vi "Main 2.3.vi"() -> ()   [LabVIEW 2022 SP3]
uses:
  <vilib>/MakerHub/LINX/Public/Utilities/Open Serial.vi
  <vilib>/MakerHub/LINX/Public/Sensors/Motion/Servo/Servo Open One Channel.vi
  Global 2 Horizontal old.vi
  Global 2 Horizontal.vi
  Global 4 Gripper old.vi
  Global 4 Gripper.vi
  Global 3 Vertical old.vi
  Global 3 Vertical.vi
  <vilib>/MakerHub/LINX/Public/Sensors/Motion/Servo/Servo Set Pulse Width One Channel.vi
  <vilib>/MakerHub/LINX/Public/Sensors/Motion/Servo/Servo Close One Channel.vi
  Global distance.vi
  Global 1 Base.vi
  Global 5 grid number.vi
  Global 6 Bool.vi
  Reading Red.vi
  Global Red Initial.vi
  Reading Green.vi
  Global Green Initial.vi
  Reading Blue.vi
  Global Blue Initial.vi
  Global Blue After Box.vi
  Global Green After Box.vi
  Global Red After Box.vi
  Colour Output.vi
  <vilib>/MakerHub/LINX/LMH-LINX.lvlib
  <vilib>/MakerHub/LINX/Public/Sensors/Motion/Servo/Servo.lvlib
panel:
  out "Numeric 6":dbl
  out "Numeric 5":dbl
  out "Numeric 4":dbl
  out "Numeric 3":dbl
  out "Numeric 2":dbl
  out "Numeric":dbl
  out "String":string
  out "Distance to Box 2":dbl
  out "Waveform Chart":dynamicdata(graph)
  out "Object detected":bool=TRUE
  out "Object not detected / Unreachable":bool=TRUE
  out "Base":i32
  out "Gripper":i32
  out "Vertical":i32
  out "Horzontal":i32
  out "Grid No":i32
  out "Starting":bool=TRUE
  out "Waiting":bool
  out "Over":bool=TRUE
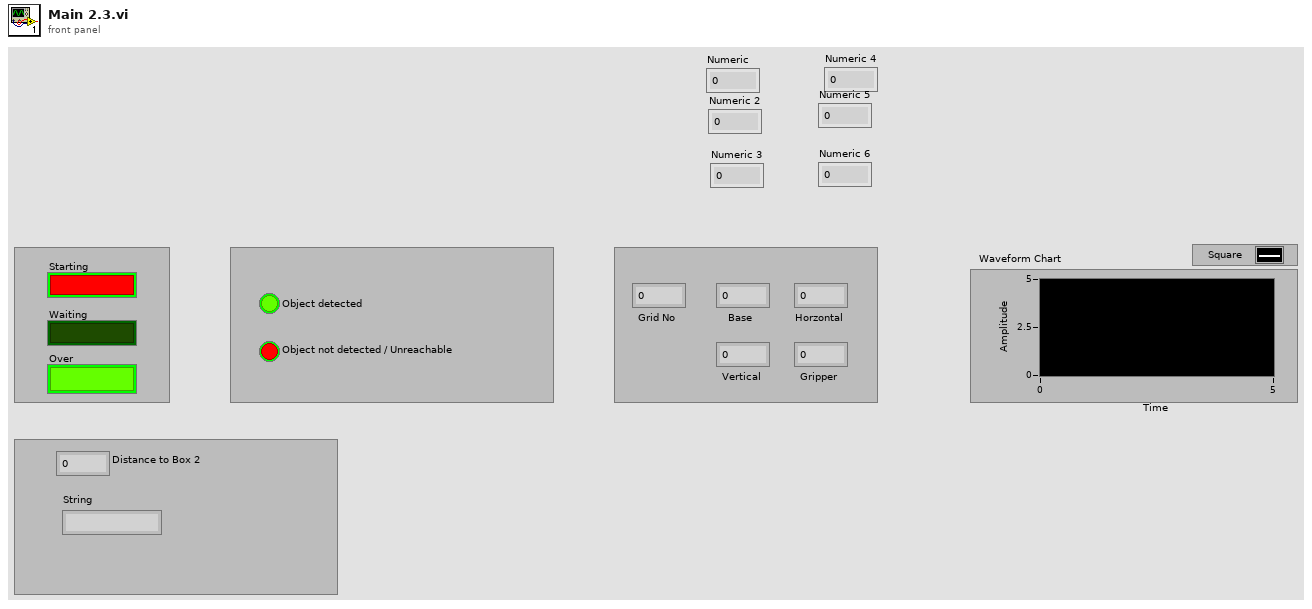
[diagram p1: front panel]
types:
  T1 = typedef "LMH-LINX.lvlib/LINX Ref.ctl" = cluster{"IO":T2, "Interface":T3, "LINX Device Config":T4}
  T2 = typedef "LMH-LINX.lvlib/Platform.ctl" = enum16{"Remote", "Local"}
  T3 = typedef "LMH-LINX.lvlib/Interface.ctl" = enum16{"Serial", "TCP"}
  T4 = typedef "LMH-LINX.lvlib/Device.lvlib/LINX Device Config.ctl" = cluster{"Interface":T3, "COM Port":refnum<visa-resource-name>, "TCP Configuration":T5, "Device Family":u8, "Device ID":u8, "Device Name":string, "TCP Ref":refnum<k5>, "Channels":T6}
  T5 = typedef "LMH-LINX.lvlib/Device.lvlib/TCP Config.ctl" = cluster{"IP Address":string, "Port":u16}
  T6 = typedef "LMH-LINX.lvlib/Channels.ctl" = cluster{"DI":u8[], "DO":u8[], "AI":u8[], "AO":u8[], "PWM":u8[], "QE":u8[], "UART":u8[], "I2C 2":u8[], "SPI":u8[], "CAN":u8[], "Servo":u8[], "AI Ref (V)":dbl, "AI Resolution (Bits)":u8, "AO Ref (V)":dbl, "AO Resolution (Bits)":u8}
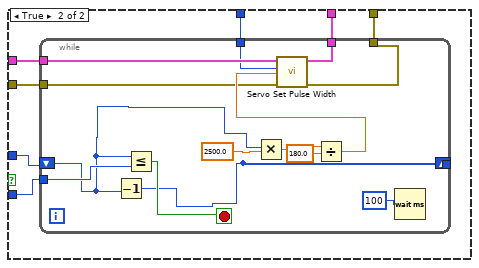
[diagram p2: hidden frame]
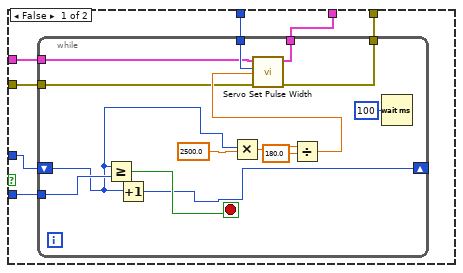
[diagram p3: hidden frame]
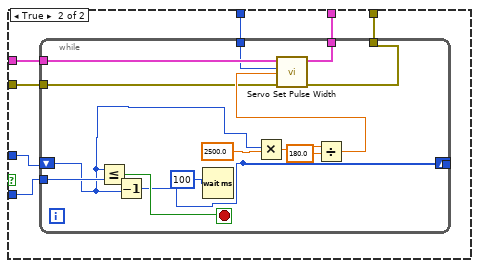
[diagram p4: hidden frame]
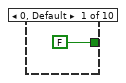
[diagram p5: hidden frame]
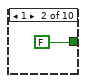
[diagram p6: hidden frame]
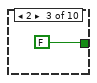
[diagram p7: hidden frame]
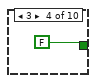
[diagram p8: hidden frame]
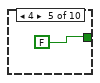
[diagram p9: hidden frame]
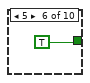
[diagram p10: hidden frame]
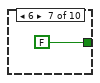
[diagram p11: hidden frame]
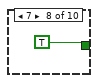
[diagram p12: hidden frame]
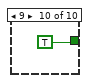
[diagram p13: hidden frame]
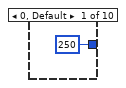
[diagram p14: hidden frame]
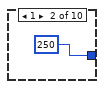
[diagram p15: hidden frame]
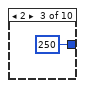
[diagram p16: hidden frame]
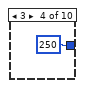
[diagram p17: hidden frame]
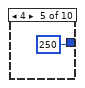
[diagram p18: hidden frame]
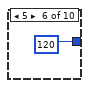
[diagram p19: hidden frame]
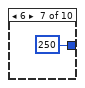
[diagram p20: hidden frame]
diagram:
  w8 = 11
  w6 = 10
  w3 = 9
  n1 = call-poly <vilib>:"Open.vi"("Serial Port"=refnum<visa-resource-name> "COM6") -> ("Error Out"=w9:errorcluster, "LINX Resource"=w10:T1)  [unwired: 8 in, 1 out]
  n2 = call-poly <vilib>:"Servo Open.vi"("Error In"=w9, "Servo Channel"=w3, "LINX Resource"=w10) -> ("Error Out"=w27:errorcluster, "LINX Resource"=w29:T1)  [unwired: 7 in]
  n3 = call-poly <vilib>:"Servo Open.vi"("Error In"=w9, "Servo Channel"=w6, "LINX Resource"=w10) -> ("Error Out"=w1:errorcluster, "LINX Resource"=w16:T1)  [unwired: 7 in]
  n4 = call-poly <vilib>:"Servo Open.vi"("Error In"=w9, "Servo Channel"=w8, "LINX Resource"=w10) -> ("Error Out"=w12:errorcluster, "LINX Resource"=w13:T1)  [unwired: 7 in]
  n5 = while {
    tunnel: w29 -> [w46]
    tunnel: [w44] -> w28
    tunnel: w27 -> [w48]
    tunnel: [w45] -> w26
    tunnel: w3 -> [w49]
    tunnel: w16 -> [w53]
    tunnel: [w52] -> w15
    tunnel: [w42] -> w14
    tunnel: w13 -> [w40]
    tunnel: w12 -> [w39]
    tunnel: [w41] -> w11
    tunnel: w8 -> [w43]
    tunnel: [w43] -> w7
    tunnel: w6 -> [w54]
    tunnel: [w54] -> w5
    tunnel: [w49] -> w4
    tunnel: [w51] -> w2
    tunnel: w1 -> [w50]
    stop <- w37 stop-if-true
    # "Arm servo control"
    n6 = global read "Global 2 Horizontal old.vi" "Numeric"() -> (w32:i32)
    n7 = global read "Global 2 Horizontal.vi" "Numeric"() -> (w31:i32)
    n8 = global read "Global 3 Vertical old.vi" "Numeric"() -> (w34:i32)
    n9 = global read "Global 3 Vertical.vi" "Numeric"() -> (w33:i32)
    n10 = global read "Global 4 Gripper old.vi" "Numeric"() -> (w36:i32)
    n11 = global read "Global 4 Gripper.vi" "Numeric"() -> (w35:i32)
    n12 = Greater?(x=w32, y=w31) -> (0:w47:bool)
    n13 = case shown="True" w47 {
      tunnel: w32 -> [w103 w124]
      tunnel: w31 -> [w104 w125]
      tunnel: w49 -> [w102 w121]
      tunnel: [w101 w123] -> w45
      tunnel: w48 -> [w100 w122]
      tunnel: w46 -> [w99 w119]
      tunnel: [w98 w120] -> w44
      frame False {
        n14 = while {
          tunnel: w104 -> [w115]
          shift-right: [w116] -> _
          shift-left: w103 -> [w108]
          tunnel: w102 -> [w110]
          tunnel: [w109] -> w98
          tunnel: [w107] -> w101
          tunnel: w100 -> [w106]
          tunnel: w99 -> [w105]
          stop <- w118 stop-if-true
          n15 = Greater Or Equal?(x=w108, y=w115) -> (x >= y?=w118:bool)
          n16 = Increment(x=w108) -> (x+1=w116:i32)
          n17 = Multiply(x=w108, y=2500.0) -> (x*y=w113:dbl)
          n18 = Divide(x=w113, y=180.0) -> (x/y=w114:dbl)
          n19 = call-poly <vilib>:"Servo Set Pulse Width.vi"("Error In"=w106, "Pulse Width (uS)"=w114, "Servo Channel"=w110, "LINX Resource"=w105) -> ("Error Out"=w107:errorcluster, "LINX Resource"=w109:T1)  [unwired: 6 in]
          n20 = Wait (ms)(milliseconds to wait=u32 100 ("millisecond timer value")) -> ()  [unwired: 1 out]
        }
      }
      frame True {
        n21 = while {
          tunnel: w125 -> [w139]
          tunnel: [w138] -> _
          shift-right: [w128] -> _
          shift-left: w124 -> [w130]
          tunnel: [w128] -> _
          tunnel: [w132] -> w123
          tunnel: w122 -> [w131]
          tunnel: w121 -> [w129]
          tunnel: [w127] -> w120
          tunnel: w119 -> [w126]
          stop <- w138 stop-if-true
          n22 = Less Or Equal?(x=w130, y=w139) -> (x <= y?=w138:bool)
          n23 = Decrement(x=w130) -> (x-1=w128:i32)
          n24 = Multiply(x=w130, y=2500.0) -> (x*y=w135:dbl)
          n25 = Divide(x=w135, y=180.0) -> (x/y=w136:dbl)
          n26 = call-poly <vilib>:"Servo Set Pulse Width.vi"("Error In"=w131, "Pulse Width (uS)"=w136, "Servo Channel"=w129, "LINX Resource"=w126) -> ("Error Out"=w132:errorcluster, "LINX Resource"=w127:T1)  [unwired: 6 in]
          n27 = Wait (ms)(milliseconds to wait=u32 100 ("millisecond timer value")) -> ()  [unwired: 1 out]
        }
      }
    }
    n28 = Greater?(x=w34, y=w33) -> (0:w55:bool)
    n29 = Greater?(x=w36, y=w35) -> (0:w38:bool)
    n30 = case shown="False" w55 {
      tunnel: w34 -> [w145 w166]
      tunnel: w33 -> [w146 w167]
      tunnel: w54 -> [w144 w161]
      tunnel: w53 -> [w143 w163]
      tunnel: [w142 w164] -> w52
      tunnel: [w141 w165] -> w51
      tunnel: w50 -> [w140 w162]
      frame False {
        n31 = while {
          tunnel: w146 -> [w157]
          shift-right: [w158] -> _
          shift-left: w145 -> [w149]
          tunnel: w144 -> [w152]
          tunnel: w143 -> [w151]
          tunnel: [w150] -> w142
          tunnel: [w148] -> w141
          tunnel: w140 -> [w147]
          stop <- w160 stop-if-true
          n32 = Greater Or Equal?(x=w149, y=w157) -> (x >= y?=w160:bool)
          n33 = Increment(x=w149) -> (x+1=w158:i32)
          n34 = Wait (ms)(milliseconds to wait=u32 100 ("millisecond timer value")) -> ()  [unwired: 1 out]
          n35 = Multiply(x=w149, y=2500.0) -> (x*y=w155:dbl)
          n36 = Divide(x=w155, y=180.0) -> (x/y=w156:dbl)
          n37 = call-poly <vilib>:"Servo Set Pulse Width.vi"("Error In"=w147, "Pulse Width (uS)"=w156, "Servo Channel"=w152, "LINX Resource"=w151) -> ("Error Out"=w148:errorcluster, "LINX Resource"=w150:T1)  [unwired: 6 in]
        }
      }
      frame True {
        n38 = while {
          tunnel: w167 -> [w181]
          shift-right: [w178] -> _
          shift-left: w166 -> [w169]
          tunnel: [w178] -> _
          tunnel: [w173] -> w165
          tunnel: [w172] -> w164
          tunnel: w163 -> [w171]
          tunnel: w162 -> [w170]
          tunnel: w161 -> [w168]
          stop <- w180 stop-if-true
          n39 = Less Or Equal?(x=w169, y=w181) -> (x <= y?=w180:bool)
          n40 = Decrement(x=w169) -> (x-1=w178:i32)
          n41 = Wait (ms)(milliseconds to wait=u32 100 ("millisecond timer value")) -> ()  [unwired: 1 out]
          n42 = Multiply(x=w169, y=2500.0) -> (x*y=w176:dbl)
          n43 = Divide(x=w176, y=180.0) -> (x/y=w177:dbl)
          n44 = call-poly <vilib>:"Servo Set Pulse Width.vi"("Error In"=w170, "Pulse Width (uS)"=w177, "Servo Channel"=w168, "LINX Resource"=w171) -> ("Error Out"=w173:errorcluster, "LINX Resource"=w172:T1)  [unwired: 6 in]
        }
      }
    }
    n45 = case shown="False" w38 {
      tunnel: w36 -> [w61 w82]
      tunnel: w35 -> [w62 w83]
      tunnel: w43 -> [w60 w77]
      tunnel: w40 -> [w59 w79]
      tunnel: [w58 w80] -> w42
      tunnel: [w57 w81] -> w41
      tunnel: w39 -> [w56 w78]
      frame False {
        n46 = while {
          tunnel: w62 -> [w73]
          shift-right: [w74] -> _
          shift-left: w61 -> [w65]
          tunnel: w60 -> [w68]
          tunnel: w59 -> [w67]
          tunnel: [w66] -> w58
          tunnel: [w64] -> w57
          tunnel: w56 -> [w63]
          stop <- w76 stop-if-true
          n47 = Greater Or Equal?(x=w65, y=w73) -> (x >= y?=w76:bool)
          n48 = Increment(x=w65) -> (x+1=w74:i32)
          n49 = Multiply(x=w65, y=2500.0) -> (x*y=w71:dbl)
          n50 = Divide(x=w71, y=180.0) -> (x/y=w72:dbl)
          n51 = call-poly <vilib>:"Servo Set Pulse Width.vi"("Error In"=w63, "Pulse Width (uS)"=w72, "Servo Channel"=w68, "LINX Resource"=w67) -> ("Error Out"=w64:errorcluster, "LINX Resource"=w66:T1)  [unwired: 6 in]
          n52 = Wait (ms)(milliseconds to wait=u32 100 ("millisecond timer value")) -> ()  [unwired: 1 out]
        }
      }
      frame True {
        n53 = while {
          tunnel: w83 -> [w97]
          shift-right: [w94] -> _
          shift-left: w82 -> [w85]
          tunnel: [w94] -> _
          tunnel: [w89] -> w81
          tunnel: [w88] -> w80
          tunnel: w79 -> [w87]
          tunnel: w78 -> [w86]
          tunnel: w77 -> [w84]
          stop <- w96 stop-if-true
          n54 = Decrement(x=w85) -> (x-1=w94:i32)
          n55 = Less Or Equal?(x=w85, y=w97) -> (x <= y?=w96:bool)
          n56 = Multiply(x=w85, y=2500.0) -> (x*y=w92:dbl)
          n57 = Divide(x=w92, y=180.0) -> (x/y=w93:dbl)
          n58 = call-poly <vilib>:"Servo Set Pulse Width.vi"("Error In"=w86, "Pulse Width (uS)"=w93, "Servo Channel"=w84, "LINX Resource"=w87) -> ("Error Out"=w89:errorcluster, "LINX Resource"=w88:T1)  [unwired: 6 in]
          n59 = Wait (ms)(milliseconds to wait=u32 100 ("millisecond timer value")) -> ()  [unwired: 1 out]
        }
      }
    }
    n60 = local read "Over"() -> (w37:bool)
  }
  n61 = call-poly <vilib>:"Servo Close.vi"("Error In"=w26, "Servo Channel"=w4, "LINX Resource"=w28) -> ("Error Out"=w23:errorcluster, "LINX Resource"=w24:T1)  [unwired: 7 in]
  n62 = call-poly <vilib>:"Servo Close.vi"("Error In"=w2, "Servo Channel"=w5, "LINX Resource"=w15) -> ("Error Out"=w20:errorcluster, "LINX Resource"=w21:T1)  [unwired: 7 in]
  n63 = call-poly <vilib>:"Servo Close.vi"("Error In"=w11, "Servo Channel"=w7, "LINX Resource"=w14) -> ("Error Out"=w17:errorcluster, "LINX Resource"=w18:T1)  [unwired: 7 in]
  n64 = call <vilib>:"Close.vi"("Error In"=w23, "LINX Resource"=w24) -> ("Error Out"=w25:errorcluster)  [unwired: 9 in]
  n65 = call <vilib>:"Close.vi"("Error In"=w20, "LINX Resource"=w21) -> ("Error Out"=w22:errorcluster)  [unwired: 9 in]
  n66 = call <vilib>:"Close.vi"("Error In"=w17, "LINX Resource"=w18) -> ("Error Out"=w19:errorcluster)  [unwired: 9 in]
  n67 = call <vilib>:"Simple Error Handler.vi"("error in (no error)"=w25) -> ()  [unwired: 4 in, 5 out]
  n68 = call <vilib>:"Simple Error Handler.vi"("error in (no error)"=w19) -> ()  [unwired: 4 in, 5 out]
  n69 = call <vilib>:"Simple Error Handler.vi"("error in (no error)"=w22) -> ()  [unwired: 4 in, 5 out]
  n70 = while {
    stop <- w184 stop-if-true
    # "Base servo control"
    # "Amplitude"
    # "Frequency"
    # "Offset"
    n71 = global read "Global 1 Base.vi" "Numeric"() -> (w183:i32)
    n72 = Divide(x=w183, y=36) -> (x/y=w192:dbl)
    n73 = Add(x=w192, y=5.0) -> (x+y=w191:dbl)
    n74 = call "Simulate Signal"("Offset"=2.5, "Duty Cycle (%)"=w191, "Frequency"=50.0, "Amplitude"=2.5) -> ("Square"=w182:dynamicdata)  [unwired: 10 in, 1 out]
    "Waveform Chart" <- w182
    n75 = call "DAQ Assistant"("data"=w182, "timeout (s)"=5.0) -> ()  [unwired: 15 in, 3 out]
    n76 = local read "Over"() -> (w184:bool)
  }
  n77 = while {
    stop <- w194 stop-if-true
    # "Ultrasonic sensor"
    n78 = global read "Global distance.vi" "Numeric"() -> (→"Distance to Box 2":dbl)
    n79 = call "ultrasonic.vi"() -> ()  [unwired: 12 in]
    n80 = local read "Over"() -> (w194:bool)
  }
  n81 = flat-sequence {
    frame #0 {
      # "Initiate"
      n82 = global write "Global 1 Base.vi" "Numeric"(250 ("Numeric")) -> ()
      n83 = global write "Global distance.vi" "Numeric"(0.0 ("Numeric")) -> ()
      n84 = global write "Global 4 Gripper.vi" "Numeric"(60 ("Numeric")) -> ()
      n85 = global write "Global 2 Horizontal.vi" "Numeric"(50 ("Numeric")) -> ()
      n86 = global write "Global 3 Vertical.vi" "Numeric"(160 ("Numeric")) -> ()
      n87 = Wait (ms)(milliseconds to wait=u32 3000 ("millisecond timer value")) -> ()  [unwired: 1 out]
      "Object not detected / Unreachable" <- FALSE
      "Object detected" <- FALSE
      "Over" <- FALSE
      "Waiting" <- FALSE
      "Starting" <- TRUE
    }
    frame #1 {
      # "Initial position"
      n88 = global write "Global 3 Vertical.vi" "Numeric"(160 ("Numeric")) -> ()
      n89 = global write "Global 4 Gripper.vi" "Numeric"(50 ("Numeric")) -> ()
      n90 = global write "Global 1 Base.vi" "Numeric"(250 ("Numeric")) -> ()
      n91 = global write "Global 2 Horizontal.vi" "Numeric"(60 ("Numeric")) -> ()
      n92 = local write "Starting"(FALSE) -> ()
      n93 = Wait (ms)(milliseconds to wait=u32 5000 ("millisecond timer value")) -> ()  [unwired: 1 out]
    }
    frame #2 {
      n94 = global read "Global 4 Gripper.vi" "Numeric"() -> (w213:i32)
      n95 = global read "Global 2 Horizontal.vi" "Numeric"() -> (w215:i32)
      n96 = global read "Global 3 Vertical.vi" "Numeric"() -> (w214:i32)
      n97 = global write "Global 2 Horizontal old.vi" "Numeric"(w215) -> ()
      n98 = global write "Global 3 Vertical old.vi" "Numeric"(w214) -> ()
      n99 = global write "Global 4 Gripper old.vi" "Numeric"(w213) -> ()
      n100 = Wait (ms)(milliseconds to wait=u32 1000 ("millisecond timer value")) -> ()  [unwired: 1 out]
    }
    frame #3 {
      # "Ready position"
      n101 = global write "Global 2 Horizontal.vi" "Numeric"(90 ("Numeric")) -> ()
      n102 = Wait (ms)(milliseconds to wait=u32 3000 ("millisecond timer value")) -> ()  [unwired: 1 out]
    }
    frame #4 {
      n103 = global write "Global 3 Vertical.vi" "Numeric"(120 ("Numeric")) -> ()
      n104 = Wait (ms)(milliseconds to wait=u32 3000 ("millisecond timer value")) -> ()  [unwired: 1 out]
    }
    frame #5 {
      n105 = global read "Global 2 Horizontal.vi" "Numeric"() -> (w222:i32)
      n106 = global read "Global 3 Vertical.vi" "Numeric"() -> (w221:i32)
      n107 = global write "Global 2 Horizontal old.vi" "Numeric"(w222) -> ()
      n108 = global write "Global 3 Vertical old.vi" "Numeric"(w221) -> ()
      n109 = Wait (ms)(milliseconds to wait=u32 1000 ("millisecond timer value")) -> ()  [unwired: 1 out]
    }
    frame #6 {
      # "Run .py"
      n110 = Open Python Session(python version="3.9" ("Python version"), python path=path "C:/Users/ASUS/AppData/Local/Programs/Python/Python39/python.exe" ("Python path")) -> (session out=w225:refnum<k35>, error out=w224:errorcluster)  [unwired: 1 in]
      n111 = node "Python Node"(w225, path "C:/Users/ASUS/Desktop/Project/grid.py" ("module path"), "detect_grid" ("function name"), w224) -> (w228:refnum<k35>, w227:errorcluster)  [unwired: 2 in, 2 out]
      n112 = Close Python Session(session in=w228, error in=w227) -> ()  [unwired: 1 out]
    }
    frame #7 {
      # "Read grid no. from .txt"
      n113 = Read from Text File(file (use dialog)=path "C:/Users/ASUS/Desktop/Project/grid_value.txt") -> (text=w232:string)  [unwired: 3 in, 3 out]
      n114 = Fract/Exp String To Number(string=w232) -> (number=w231:dbl)  [unwired: 3 in, 1 out]
      "Grid No" <- w231
      n115 = global write "Global 5 grid number.vi" "Numeric"(w231) -> ()
    }
    frame #8 {
      # "Grid selection"
      n116 = global read "Global 5 grid number.vi" "Numeric"() -> (w236:i32)
      n117 = case shown="8" w236 {
        tunnel: [FALSE FALSE FALSE FALSE FALSE TRUE FALSE TRUE FALSE TRUE] -> w235
        frame 0, Default {
        }
        frame 1 {
        }
        frame 2 {
        }
        frame 3 {
        }
        frame 4 {
        }
        frame 5 {
        }
        frame 6 {
        }
        frame 7 {
        }
        frame 8 {
        }
        frame 9 {
        }
      }
      n118 = global write "Global 6 Bool.vi" "Boolean"(w235) -> ()
      n119 = Wait (ms)(milliseconds to wait=u32 3000 ("millisecond timer value")) -> ()  [unwired: 1 out]
    }
    frame #9 {
      n120 = global read "Global 6 Bool.vi" "Boolean"() -> (w248:bool)
      n121 = Not(x=w248) -> (.not. x?=w247:bool)
      n122 = local write "Object not detected / Unreachable"(w247) -> ()
      n123 = local write "Object detected"(w248) -> ()
    }
    frame #10 {
      # "Get angles"
      n124 = global read "Global 5 grid number.vi" "Numeric"() -> (w251:i32)
      n125 = case shown="7" w251 {
        tunnel: [250 250 250 250 250 120 250 160 250 65] -> w250
        frame 0, Default {
        }
        frame 1 {
        }
        frame 2 {
        }
        frame 3 {
        }
        frame 4 {
        }
        frame 5 {
        }
        frame 6 {
        }
        frame 7 {
        }
        frame 8 {
        }
        frame 9 {
        }
      }
      "Base" <- w250
      n126 = global write "Global 1 Base.vi" "Numeric"(w250) -> ()
      n127 = Wait (ms)(milliseconds to wait=u32 3000 ("millisecond timer value")) -> ()  [unwired: 1 out]
    }
    frame #11 {
      # "Get angles"
      n128 = global read "Global 5 grid number.vi" "Numeric"() -> (w263:i32)
      n129 = case shown="8" w263 {
        tunnel: [0 0 0 0 0 120 0 120 0 120] -> w264
        frame 0, Default {
        }
        frame 1 {
        }
        frame 2 {
        }
        frame 3 {
        }
        frame 4 {
        }
        frame 5 {
        }
        frame 6 {
        }
        frame 7 {
        }
        frame 8 {
        }
        frame 9 {
        }
      }
      "Gripper" <- w264
      n130 = global write "Global 4 Gripper.vi" "Numeric"(w264) -> ()
      n131 = Wait (ms)(milliseconds to wait=u32 3000 ("millisecond timer value")) -> ()  [unwired: 1 out]
    }
    frame #12 {
      n132 = global read "Global 4 Gripper.vi" "Numeric"() -> (w275:i32)
      n133 = global write "Global 4 Gripper old.vi" "Numeric"(w275) -> ()
    }
    frame #13 {
      # "Get angles"
      n134 = global read "Global 5 grid number.vi" "Numeric"() -> (w278:i32)
      n135 = case shown="8" w278 {
        tunnel: [160 160 160 160 160 150 160 140 160 140] -> w277
        frame 0, Default {
        }
        frame 1 {
        }
        frame 2 {
        }
        frame 3 {
        }
        frame 4 {
        }
        frame 5 {
        }
        frame 6 {
        }
        frame 7 {
        }
        frame 8 {
        }
        frame 9 {
        }
      }
      "Vertical" <- w277
      n136 = global write "Global 3 Vertical.vi" "Numeric"(w277) -> ()
      n137 = Wait (ms)(milliseconds to wait=u32 3000 ("millisecond timer value")) -> ()  [unwired: 1 out]
    }
    frame #14 {
      n138 = global read "Global 3 Vertical.vi" "Numeric"() -> (w289:i32)
      n139 = global write "Global 3 Vertical old.vi" "Numeric"(w289) -> ()
    }
    frame #15 {
      # "Get angles"
      n140 = global read "Global 5 grid number.vi" "Numeric"() -> (w291:i32)
      n141 = case shown="9" w291 {
        tunnel: [60 60 60 60 60 125 60 118 60 115] -> w292
        frame 0, Default {
        }
        frame 1 {
        }
        frame 2 {
        }
        frame 3 {
        }
        frame 4 {
        }
        frame 5 {
        }
        frame 6 {
        }
        frame 7 {
        }
        frame 8 {
        }
        frame 9 {
        }
      }
      "Horzontal" <- w292
      n142 = global write "Global 2 Horizontal.vi" "Numeric"(w292) -> ()
      n143 = Wait (ms)(milliseconds to wait=u32 3000 ("millisecond timer value")) -> ()  [unwired: 1 out]
    }
    frame #16 {
      n144 = global read "Global 2 Horizontal.vi" "Numeric"() -> (w304:i32)
      n145 = global write "Global 2 Horizontal old.vi" "Numeric"(w304) -> ()
      n146 = Wait (ms)(milliseconds to wait=u32 3000 ("millisecond timer value")) -> ()  [unwired: 1 out]
    }
    frame #17 {
      n147 = global read "Global 6 Bool.vi" "Boolean"() -> (w305:bool)
      n148 = case shown="False" w305 {
        frame False {
          n149 = flat-sequence {
            frame #0 {
              n150 = global read "Global 6 Bool.vi" "Boolean"() -> (w306:bool)
              n151 = local write "Object not detected / Unreachable"(w306) -> ()
            }
            frame #1 {
              n152 = local write "Waiting"(TRUE) -> ()
              n153 = Wait (ms)(milliseconds to wait=u32 10000) -> ()  [unwired: 1 out]
            }
            frame #2 {
              n154 = call "Buzzer.vi"() -> ()  [unwired: 12 in]
            }
            frame #3 {
              n155 = local write "Waiting"(FALSE) -> ()
              n156 = Wait (ms)(milliseconds to wait=u32 3000) -> ()  [unwired: 1 out]
              n157 = local write "Over"(TRUE) -> ()
            }
          }
        }
        frame True {
          n158 = flat-sequence {
            frame #0 {
              # "Close the gripper"
              n159 = global write "Global 4 Gripper.vi" "Numeric"(50) -> ()
              n160 = Wait (ms)(milliseconds to wait=u32 5000) -> ()  [unwired: 1 out]
            }
            frame #1 {
              n161 = global read "Global 4 Gripper.vi" "Numeric"() -> (w315:i32)
              n162 = global write "Global 4 Gripper old.vi" "Numeric"(w315) -> ()
              n163 = Wait (ms)(milliseconds to wait=u32 5000) -> ()  [unwired: 1 out]
            }
            frame #2 {
              n164 = global write "Global 2 Horizontal.vi" "Numeric"(65) -> ()
              n165 = Wait (ms)(milliseconds to wait=u32 5000 ("millisecond timer value")) -> ()  [unwired: 1 out]
            }
            frame #3 {
              # "Pick up the box"
              n166 = global write "Global 3 Vertical.vi" "Numeric"(170) -> ()
              n167 = Wait (ms)(milliseconds to wait=u32 5000 ("millisecond timer value")) -> ()  [unwired: 1 out]
            }
            frame #4 {
              n168 = global read "Global 2 Horizontal.vi" "Numeric"() -> (w322:i32)
              n169 = global read "Global 3 Vertical.vi" "Numeric"() -> (w321:i32)
              n170 = global write "Global 2 Horizontal old.vi" "Numeric"(w322) -> ()
              n171 = global write "Global 3 Vertical old.vi" "Numeric"(w321) -> ()
              n172 = Wait (ms)(milliseconds to wait=u32 2000 ("millisecond timer value")) -> ()  [unwired: 1 out]
            }
            frame #5 {
              n173 = call "Colour.vi"() -> ()  [unwired: 12 in]
            }
            frame #6 {
              n174 = global read "Reading Red.vi" "Numeric"() -> (w325:dbl)
              "Numeric" <- w325
              n175 = global read "Reading Green.vi" "Numeric"() -> (w324:dbl)
              "Numeric 2" <- w324
              n176 = global read "Reading Blue.vi" "Numeric"() -> (w323:dbl)
              "Numeric 3" <- w323
              n177 = global write "Global Red Initial.vi" "Numeric"(w325) -> ()
              n178 = global write "Global Green Initial.vi" "Numeric"(w324) -> ()
              n179 = global write "Global Blue Initial.vi" "Numeric"(w323) -> ()
            }
            frame #7 {
              n180 = global write "Global 1 Base.vi" "Numeric"(-70 ("Numeric")) -> ()
              n181 = Wait (ms)(milliseconds to wait=u32 1000 ("millisecond timer value")) -> ()  [unwired: 1 out]
            }
            frame #8 {
              n182 = global write "Global 3 Vertical.vi" "Numeric"(160) -> ()
              n183 = Wait (ms)(milliseconds to wait=u32 1000 ("millisecond timer value")) -> ()  [unwired: 1 out]
            }
            frame #9 {
              n184 = global read "Global 3 Vertical.vi" "Numeric"() -> (w330:i32)
              n185 = global write "Global 3 Vertical old.vi" "Numeric"(w330) -> ()
            }
            frame #10 {
              n186 = call "Colour.vi"() -> ()  [unwired: 12 in]
            }
            frame #11 {
              n187 = global read "Reading Red.vi" "Numeric"() -> (w333:dbl)
              "Numeric 4" <- w333
              n188 = global read "Reading Green.vi" "Numeric"() -> (w332:dbl)
              "Numeric 5" <- w332
              n189 = global read "Reading Blue.vi" "Numeric"() -> (w331:dbl)
              "Numeric 6" <- w331
              n190 = global write "Global Red After Box.vi" "Numeric"(w333) -> ()
              n191 = global write "Global Green After Box.vi" "Numeric"(w332) -> ()
              n192 = global write "Global Blue After Box.vi" "Numeric"(w331) -> ()
            }
            frame #12 {
              n193 = global write "Global 4 Gripper.vi" "Numeric"(50) -> ()
              n194 = Wait (ms)(milliseconds to wait=u32 5000 ("millisecond timer value")) -> ()  [unwired: 1 out]
            }
            frame #13 {
              n195 = call "ColourCheck.vi"() -> ()  [unwired: 12 in]
            }
            frame #14 {
              n196 = global read "Colour Output.vi" "String"() -> (→"String":string)
            }
            frame #15 {
              n197 = global read "Colour Output.vi" "String"() -> (w337:string)
              n198 = case shown="\"red\", Default" w337 {
                frame "red", Default {
                  n199 = flat-sequence {
                    frame #0 {
                      n200 = global write "Global 1 Base.vi" "Numeric"(-70 ("Numeric")) -> ()
                      n201 = Wait (ms)(milliseconds to wait=u32 1000 ("millisecond timer value")) -> ()  [unwired: 1 out]
                    }
                    frame #1 {
                      n202 = global write "Global 3 Vertical.vi" "Numeric"(160) -> ()
                      n203 = Wait (ms)(milliseconds to wait=u32 1000 ("millisecond timer value")) -> ()  [unwired: 1 out]
                    }
                    frame #2 {
                      n204 = Wait (ms)(milliseconds to wait=u32 5000 ("millisecond timer value")) -> ()  [unwired: 1 out]
                      n205 = global write "Global 2 Horizontal.vi" "Numeric"(110) -> ()
                    }
                    frame #3 {
                      n206 = global read "Global 2 Horizontal.vi" "Numeric"() -> (w345:i32)
                      n207 = global read "Global 3 Vertical.vi" "Numeric"() -> (w344:i32)
                      n208 = global write "Global 2 Horizontal old.vi" "Numeric"(w345) -> ()
                      n209 = global write "Global 3 Vertical old.vi" "Numeric"(w344) -> ()
                    }
                    frame #4 {
                      n210 = global write "Global 4 Gripper.vi" "Numeric"(120) -> ()
                      n211 = Wait (ms)(milliseconds to wait=u32 5000 ("millisecond timer value")) -> ()  [unwired: 1 out]
                    }
                    frame #5 {
                      n212 = global read "Global 4 Gripper.vi" "Numeric"() -> (w349:i32)
                      n213 = global write "Global 4 Gripper old.vi" "Numeric"(w349) -> ()
                      n214 = Wait (ms)(milliseconds to wait=u32 3000) -> ()  [unwired: 1 out]
                    }
                    frame #6 {
                      n215 = global write "Global 3 Vertical.vi" "Numeric"(180) -> ()
                      n216 = Wait (ms)(milliseconds to wait=u32 5000 ("millisecond timer value")) -> ()  [unwired: 1 out]
                    }
                    frame #7 {
                      n217 = Wait (ms)(milliseconds to wait=u32 5000 ("millisecond timer value")) -> ()  [unwired: 1 out]
                      n218 = global write "Global 2 Horizontal.vi" "Numeric"(70) -> ()
                    }
                    frame #8 {
                      n219 = global read "Global 2 Horizontal.vi" "Numeric"() -> (w354:i32)
                      n220 = global read "Global 3 Vertical.vi" "Numeric"() -> (w355:i32)
                      n221 = global write "Global 2 Horizontal old.vi" "Numeric"(w354) -> ()
                      n222 = global write "Global 3 Vertical old.vi" "Numeric"(w355) -> ()
                    }
                    frame #9 {
                      n223 = global write "Global 4 Gripper.vi" "Numeric"(60) -> ()
                    }
                  }
                }
                frame "green" {
                  n224 = flat-sequence {
                    frame #0 {
                      n225 = global write "Global 1 Base.vi" "Numeric"(-20 ("Numeric")) -> ()
                      n226 = Wait (ms)(milliseconds to wait=u32 1000 ("millisecond timer value")) -> ()  [unwired: 1 out]
                    }
                    frame #1 {
                      n227 = global write "Global 3 Vertical.vi" "Numeric"(160) -> ()
                      n228 = Wait (ms)(milliseconds to wait=u32 1000 ("millisecond timer value")) -> ()  [unwired: 1 out]
                    }
                    frame #2 {
                      n229 = Wait (ms)(milliseconds to wait=u32 5000 ("millisecond timer value")) -> ()  [unwired: 1 out]
                      n230 = global write "Global 2 Horizontal.vi" "Numeric"(115) -> ()
                    }
                    frame #3 {
                      n231 = global read "Global 2 Horizontal.vi" "Numeric"() -> (w365:i32)
                      n232 = global read "Global 3 Vertical.vi" "Numeric"() -> (w364:i32)
                      n233 = global write "Global 2 Horizontal old.vi" "Numeric"(w365) -> ()
                      n234 = global write "Global 3 Vertical old.vi" "Numeric"(w364) -> ()
                      n235 = Wait (ms)(milliseconds to wait=u32 1000 ("millisecond timer value")) -> ()  [unwired: 1 out]
                    }
                    frame #4 {
                      n236 = global write "Global 4 Gripper.vi" "Numeric"(120) -> ()
                      n237 = Wait (ms)(milliseconds to wait=u32 3000 ("millisecond timer value")) -> ()  [unwired: 1 out]
                    }
                    frame #5 {
                      n238 = global read "Global 4 Gripper.vi" "Numeric"() -> (w369:i32)
                      n239 = global write "Global 4 Gripper old.vi" "Numeric"(w369) -> ()
                      n240 = Wait (ms)(milliseconds to wait=u32 5000) -> ()  [unwired: 1 out]
                    }
                    frame #6 {
                      n241 = global write "Global 3 Vertical.vi" "Numeric"(180) -> ()
                      n242 = Wait (ms)(milliseconds to wait=u32 1000 ("millisecond timer value")) -> ()  [unwired: 1 out]
                    }
                    frame #7 {
                      n243 = Wait (ms)(milliseconds to wait=u32 5000 ("millisecond timer value")) -> ()  [unwired: 1 out]
                      n244 = global write "Global 2 Horizontal.vi" "Numeric"(70) -> ()
                    }
                    frame #8 {
                      n245 = global read "Global 2 Horizontal.vi" "Numeric"() -> (w375:i32)
                      n246 = global read "Global 3 Vertical.vi" "Numeric"() -> (w376:i32)
                      n247 = global write "Global 2 Horizontal old.vi" "Numeric"(w375) -> ()
                      n248 = global write "Global 3 Vertical old.vi" "Numeric"(w376) -> ()
                      n249 = Wait (ms)(milliseconds to wait=u32 1000 ("millisecond timer value")) -> ()  [unwired: 1 out]
                    }
                    frame #9 {
                      n250 = global write "Global 4 Gripper.vi" "Numeric"(60) -> ()
                      n251 = Wait (ms)(milliseconds to wait=u32 1000 ("millisecond timer value")) -> ()  [unwired: 1 out]
                    }
                  }
                }
                frame "blue" {
                  n252 = flat-sequence {
                    frame #0 {
                      n253 = global write "Global 1 Base.vi" "Numeric"(20 ("Numeric")) -> ()
                      n254 = Wait (ms)(milliseconds to wait=u32 1000 ("millisecond timer value")) -> ()  [unwired: 1 out]
                    }
                    frame #1 {
                      n255 = global write "Global 3 Vertical.vi" "Numeric"(180) -> ()
                      n256 = Wait (ms)(milliseconds to wait=u32 1000 ("millisecond timer value")) -> ()  [unwired: 1 out]
                    }
                    frame #2 {
                      n257 = Wait (ms)(milliseconds to wait=u32 5000 ("millisecond timer value")) -> ()  [unwired: 1 out]
                      n258 = global write "Global 2 Horizontal.vi" "Numeric"(125) -> ()
                    }
                    frame #3 {
                      n259 = global read "Global 2 Horizontal.vi" "Numeric"() -> (w387:i32)
                      n260 = global read "Global 3 Vertical.vi" "Numeric"() -> (w386:i32)
                      n261 = global write "Global 2 Horizontal old.vi" "Numeric"(w387) -> ()
                      n262 = global write "Global 3 Vertical old.vi" "Numeric"(w386) -> ()
                      n263 = Wait (ms)(milliseconds to wait=u32 1000 ("millisecond timer value")) -> ()  [unwired: 1 out]
                    }
                    frame #4 {
                      n264 = global write "Global 4 Gripper.vi" "Numeric"(120) -> ()
                      n265 = Wait (ms)(milliseconds to wait=u32 3000 ("millisecond timer value")) -> ()  [unwired: 1 out]
                    }
                    frame #5 {
                      n266 = global read "Global 4 Gripper.vi" "Numeric"() -> (w391:i32)
                      n267 = global write "Global 4 Gripper old.vi" "Numeric"(w391) -> ()
                      n268 = Wait (ms)(milliseconds to wait=u32 5000) -> ()  [unwired: 1 out]
                    }
                    frame #6 {
                      n269 = global write "Global 3 Vertical.vi" "Numeric"(180) -> ()
                      n270 = Wait (ms)(milliseconds to wait=u32 1000 ("millisecond timer value")) -> ()  [unwired: 1 out]
                    }
                    frame #7 {
                      n271 = Wait (ms)(milliseconds to wait=u32 5000 ("millisecond timer value")) -> ()  [unwired: 1 out]
                      n272 = global write "Global 2 Horizontal.vi" "Numeric"(70) -> ()
                    }
                    frame #8 {
                      n273 = global read "Global 2 Horizontal.vi" "Numeric"() -> (w397:i32)
                      n274 = global read "Global 3 Vertical.vi" "Numeric"() -> (w398:i32)
                      n275 = global write "Global 2 Horizontal old.vi" "Numeric"(w397) -> ()
                      n276 = global write "Global 3 Vertical old.vi" "Numeric"(w398) -> ()
                      n277 = Wait (ms)(milliseconds to wait=u32 1000 ("millisecond timer value")) -> ()  [unwired: 1 out]
                    }
                    frame #9 {
                      n278 = global write "Global 4 Gripper.vi" "Numeric"(60) -> ()
                      n279 = Wait (ms)(milliseconds to wait=u32 1000 ("millisecond timer value")) -> ()  [unwired: 1 out]
                    }
                  }
                }
              }
            }
            frame #16 {
              n280 = local write "Over"(TRUE) -> ()
              n281 = Wait (ms)(milliseconds to wait=u32 3000 ("millisecond timer value")) -> ()  [unwired: 1 out]
            }
          }
        }
      }
    }
  }
